vi "Set legs frame colors.vi"(8 "error in (no error)":errorcluster, 10 "Legs frame":u32(colorbox), 11 "Detector ref in":refnum<vi>) -> (0 "error out":errorcluster, 3 "Detector ref out":refnum<vi>)   [LabVIEW 2016]
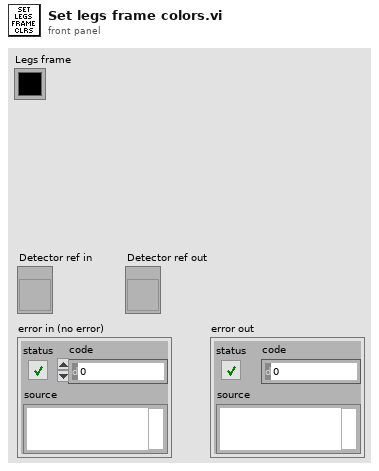
[diagram p1: front panel]
types:
  T1 = typedef "LVRGBAColorTypeDef.ctl" = cluster{"Red":sgl, "Green":sgl, "Blue":sgl, "Alpha":sgl}
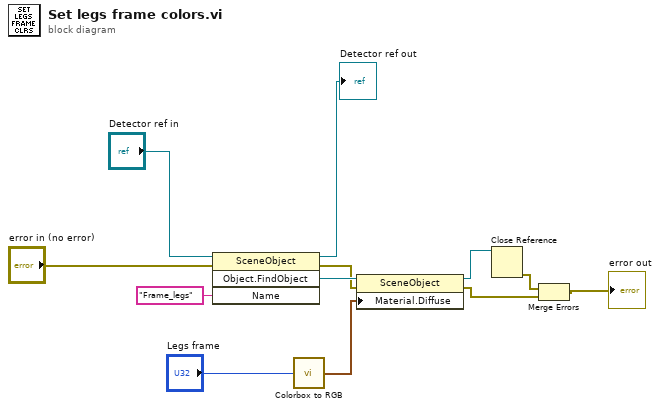
[diagram p0: block diagram]
diagram:
  n1 = invoke class="SceneObject" method="Object.FindObject"(reference="Detector ref in", error in="error in (no error)", "Name"="Frame_legs") -> (reference out=→"Detector ref out":refnum<vi>, error out=w2:errorcluster, "FindObject"=w3:refnum<vi>)  [unwired: 1 in, 1 out]
  n2 = call "Colorbox to RGB.vi"("Color"="Legs frame") -> ("Material"=w4:T1)
  n3 = property class="SceneObject"(reference=w3, error in=w2, "Material.Diffuse"=w4) -> (reference out=w6:refnum<vi>, error out=w5:errorcluster)
  n4 = Close Reference(reference=w6) -> (error out=w7:errorcluster)  [unwired: 1 in]
  n5 = Merge Errors(w7, w5) -> (→"error out":errorcluster)
